vi "Initialize MeasurementLink Session.vi"(7 "remote connection options":T2, 8 "error in":errorcluster, 9 "initialize session behavior":T1, 10 "session initialization parameters":T3, 11 "session factory in":refnum<class "Session Factory.lvclass">) -> (0 "error out":errorcluster, 2 "session out":variant, 3 "session factory out":refnum<class "Session Factory.lvclass">)   [LabVIEW 2021, in "Keysight 34461A DMM Instrument.lvlib" / "Session Factory.lvclass"]
uses:
  Session Factory.lvclass
  Session Factory.lvclass/Session Factory.ctl
  <vilib>/Plug-In SDKs/Sessions/Instrument/ISession Factory/ISession Factory.lvclass
  <vilib>/Plug-In SDKs/Sessions/Instrument/ISession Factory/Initialize and Close Session Behavior.ctl
  <instrlib>/Agilent 3446X Series/Public/Initialize.vi
  <instrlib>/Agilent 3446X Series/Agilent 3446X Series.lvlib
  Get VISA gRPC Open Close Behavior.vi
  <vilib>/NI-VISA/VISA Open for gRPC Session.vi
  <vilib>/Plug-In SDKs/Sessions/Instrument/ISession Factory/Remote Connection Options.ctl
  <vilib>/Plug-In SDKs/Sessions/Instrument/ISession Factory/Session Initialization Parameters.ctl
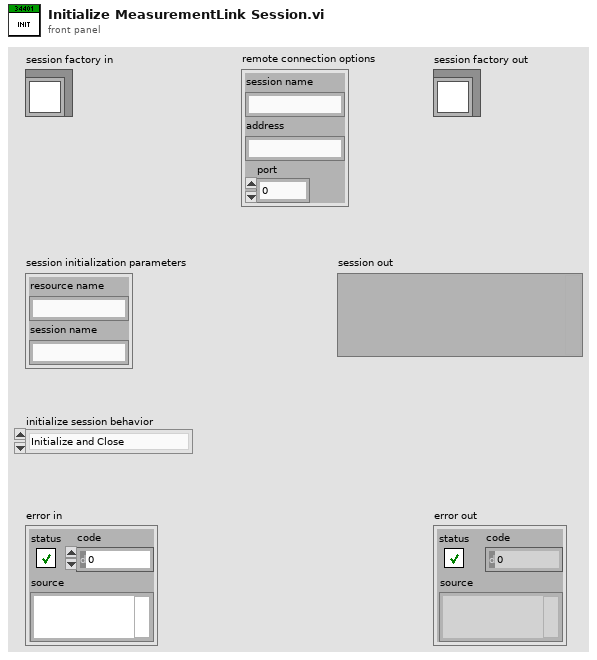
[diagram p1: front panel]
types:
  T1 = typedef "NI Session Management Instrument.lvlib/ISession Factory.lvclass/Initialize and Close Session Behavior.ctl" = enum16{"Initialize and Close", "Attach and Detach", "Initialize and Detach", "Attach and Close"}
  T2 = typedef "NI Session Management Instrument.lvlib/ISession Factory.lvclass/Remote Connection Options.ctl" = cluster{"session name":string, "address":string, "port":u32}
  T3 = typedef "NI Session Management Instrument.lvlib/ISession Factory.lvclass/Session Initialization Parameters.ctl" = cluster{"resource name":string, "session name":string}
  T4 = typedef "VISA gRPC Open Close Behavior.ctl" = enum16{"Auto", "Initialize and Close", "Attach and Detach", "Initialize and Detach", "Attach and Close"}
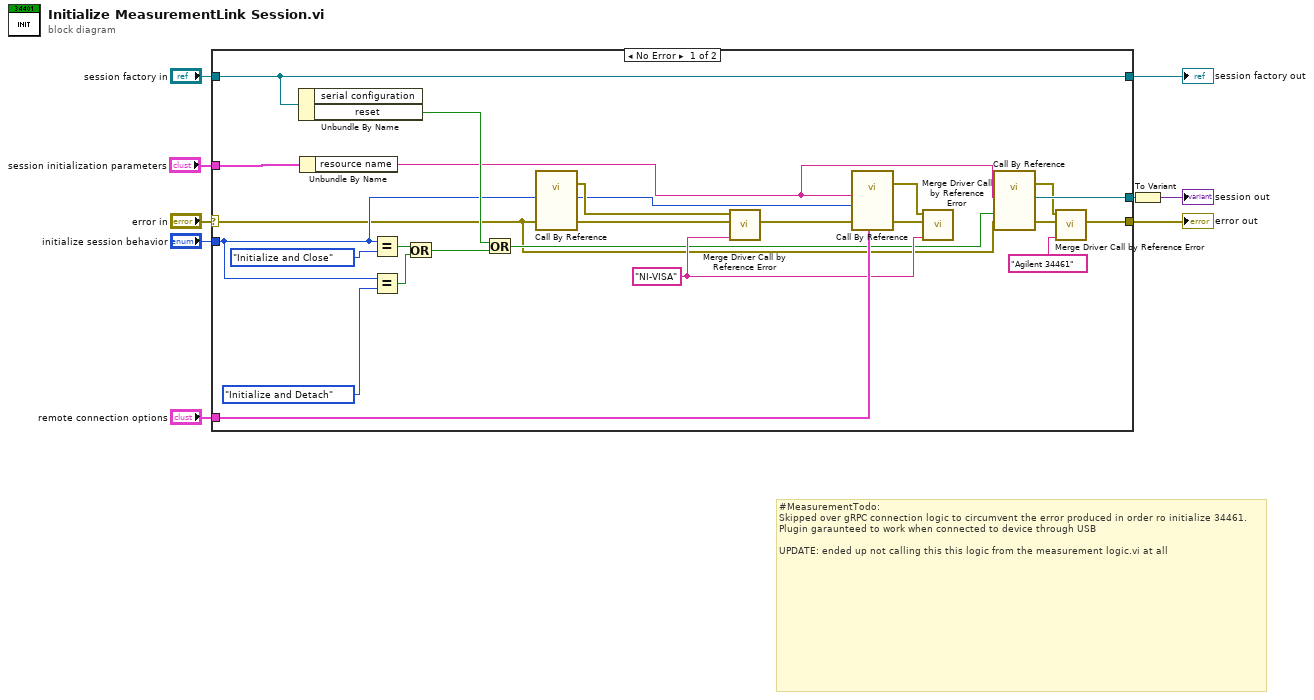
[diagram p0: block diagram]
diagram:
  # "#MeasurementTodo:\nSkipped over gRPC connection logic to circumvent the error produced in order ro initialize 34461. \nPlugin garaunteed to work when connected to device through USB\n\nUPDATE: ended up not calling this this logic from the measurement logic.vi at all"
  n1 = case shown="No Error" "error in" {
    selector: "error in" -> [w10 w35]
    tunnel: [w23 w35] -> w8
    tunnel: "session factory in" -> [w33 w36]
    tunnel: [w33 w36] -> w6
    tunnel: "initialize session behavior" -> [w22 _]
    tunnel: "session initialization parameters" -> [w34 _]
    tunnel: "remote connection options" -> [w26 _]
    tunnel: [w16 _] -> w1
    frame No Error {
      w21 = "NI-VISA" ("driver name")
      n2 = Unbundle By Name(w33) -> ("reset"=w31:bool)  [unwired: 1 out]
      n3 = Unbundle By Name(w34) -> ("resource name"=w11:string)
      n4 = Equal?(x=w22, y=Initialize_and_Close_Session_Behavior."Initialize and Close" ("initialize session behavior")) -> (x = y?=w28:bool)
      n5 = Equal?(x=w22, y=Initialize_and_Close_Session_Behavior."Initialize and Detach" ("initialize session behavior")) -> (x = y?=w27:bool)
      n6 = Or(x=w28, y=w27) -> (x .or. y?=w30:bool)
      n7 = Or(x=w31, y=w30) -> (x .or. y?=w17:bool)
      n8 = call-by-ref "?"("error in (no error)"=w10, "initialize session behavior"=w22) -> (error out=w19:errorcluster, 0:"error out"=w20:errorcluster, "open/close behavior"=w18:T4)  [unwired: 10 in, 1 out]
      n9 = call <vilib>:"Merge Driver Call by Reference Error.vi"("driver name"=w21, "called vi error"=w20, "call by ref error"=w19) -> ("error out"=w13:errorcluster)  [unwired: 8 in]
      n10 = call-by-ref "?"("gRPC Options"=w26, "error in (no error)"=w13, "Open/Close Behavior"=w18, "VISA resource name"=w11) -> (error out=w25:errorcluster, 0:"error out"=w12:errorcluster)  [unwired: 8 in, 2 out]
      n11 = call <vilib>:"Merge Driver Call by Reference Error.vi"("driver name"=w21, "called vi error"=w12, "call by ref error"=w25) -> ()  [unwired: 8 in, 1 out]
      n12 = call-by-ref "?"("error in (no error)"=w10, "Reset (True)"=w17, "VISA resource name"=w11) -> (error out=w15:errorcluster, 0:"error out"=w14:errorcluster, "VISA resource name out"=w16:refnum<visa-resource-name>)  [unwired: 9 in, 1 out]
      n13 = call <vilib>:"Merge Driver Call by Reference Error.vi"("driver name"="Agilent 34461", "called vi error"=w14, "call by ref error"=w15) -> ("error out"=w23:errorcluster)  [unwired: 8 in]
    }
    frame Error {
    }
  }
  "error out" <- w8
  "session factory out" <- w6
  n14 = To Variant(anything=w1) -> (Variant=→"session out":variant)
